vi "PadVariantArray.vi"(10 "PadBy":i32, 11 "Array In":variant) -> (1 "Array of variant values":variant[](array[variant]), 3 "Array out":variant)   [LabVIEW 2017]
uses:
  <vilib>/Utility/Data Type/NI_Data Type.lvlib
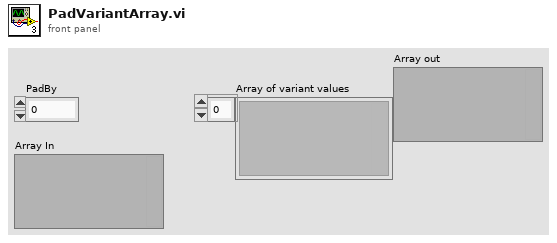
[diagram p1: front panel]
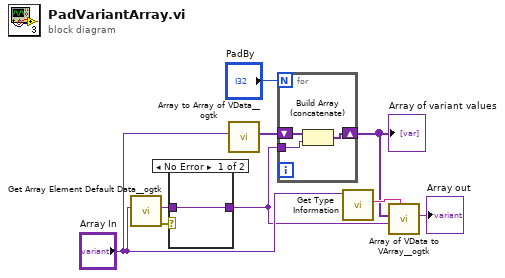
[diagram p0: block diagram]
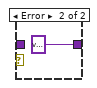
[diagram p2: hidden frame]
diagram:
  n1 = call <userlib>:"Get Array Element Default Data__ogtk.vi"("Array"="Array In") -> ("error out"=w3:errorcluster, "Array Element Default Data"=w2:variant)  [unwired: 9 in]
  n2 = case shown="No Error" w3 {
    tunnel: w2 -> [w10 _]
    tunnel: [w10 variant ("Array Element Default Data")] -> w1
    frame No Error {
    }
    frame Error {
    }
  }
  n3 = call <userlib>:"Array to Array of VData__ogtk.vi"("MultiD Array"="Array In") -> ("1D Array of Variants"=w8:variant[])  [unwired: 9 in, 1 out]
  n4 = for {
    N: "PadBy" -> [_]
    tunnel: w1 -> [w13]
    shift-right: [w12] -> w5
    shift-left: w8 -> [w14]
    n5 = Build Array (concatenate)(w14, w13) -> (w12:variant[])
  }
  "Array of variant values" <- w5
  n6 = call <vilib>:"Get Type Information.vi"("Variant"="Array In") -> ("Name"=w9:string)  [unwired: 6 in, 4 out]
  n7 = call <userlib>:"Array of VData to VArray__ogtk.vi"("Array Name"=w9, "Element Type (when empty)"=w1, "1D Array of VData"=w5) -> ("VArray"=→"Array out":variant)  [unwired: 7 in, 1 out]
